vi "test.Zorder.vi"() -> ()   [LabVIEW 2020]
uses:
  WINUTIL.LLB/Window Rectangle.ctl
  <vilib>/Utility/miscctls.llb/LVRectTypeDef.ctl
  <userlib>/_OpenG.lib/comparison/comparison.llb/Boolean Changed__ogtk.vi
  WINUTIL.LLB/WINUTIL.lvlib
panel:
  in  "topmost":bool
  in  "stop":bool
  out "Array":T1[](array[typedef])
  out "Refnum out 2":T2[](array[typedef])
  out "window name 2":string[](array[string])
  out "Front Panel Window:Panel Bounds":T3
  out "window rect":T1
  out "window name":string
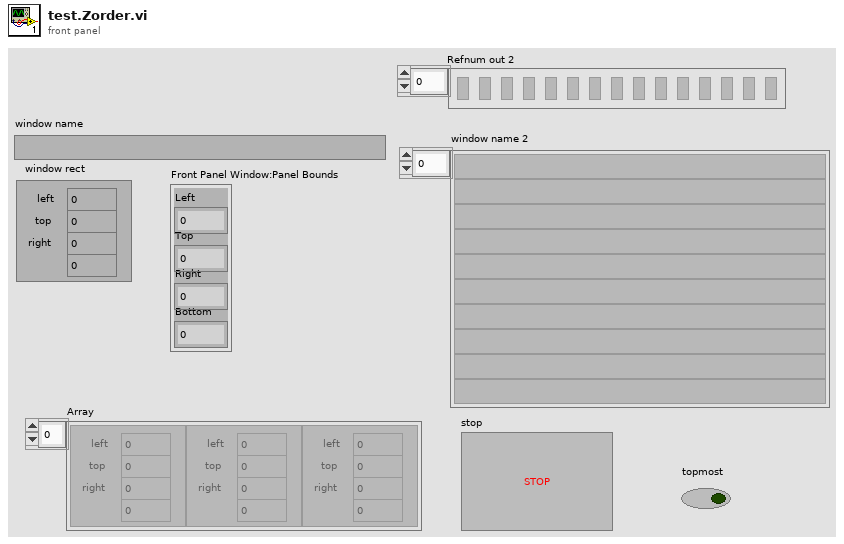
[diagram p1: front panel]
types:
  T1 = typedef "WINUTIL.lvlib/Window Rectangle.ctl" = cluster{"left":i16, "top":i16, "right":i16, "bottom":i16}
  T2 = typedef "WINUTIL.lvlib/Window Refnum" = refnum<k1>
  T3 = typedef "LVRectTypeDef.ctl" = cluster{"Left":i16, "Top":i16, "Right":i16, "Bottom":i16}
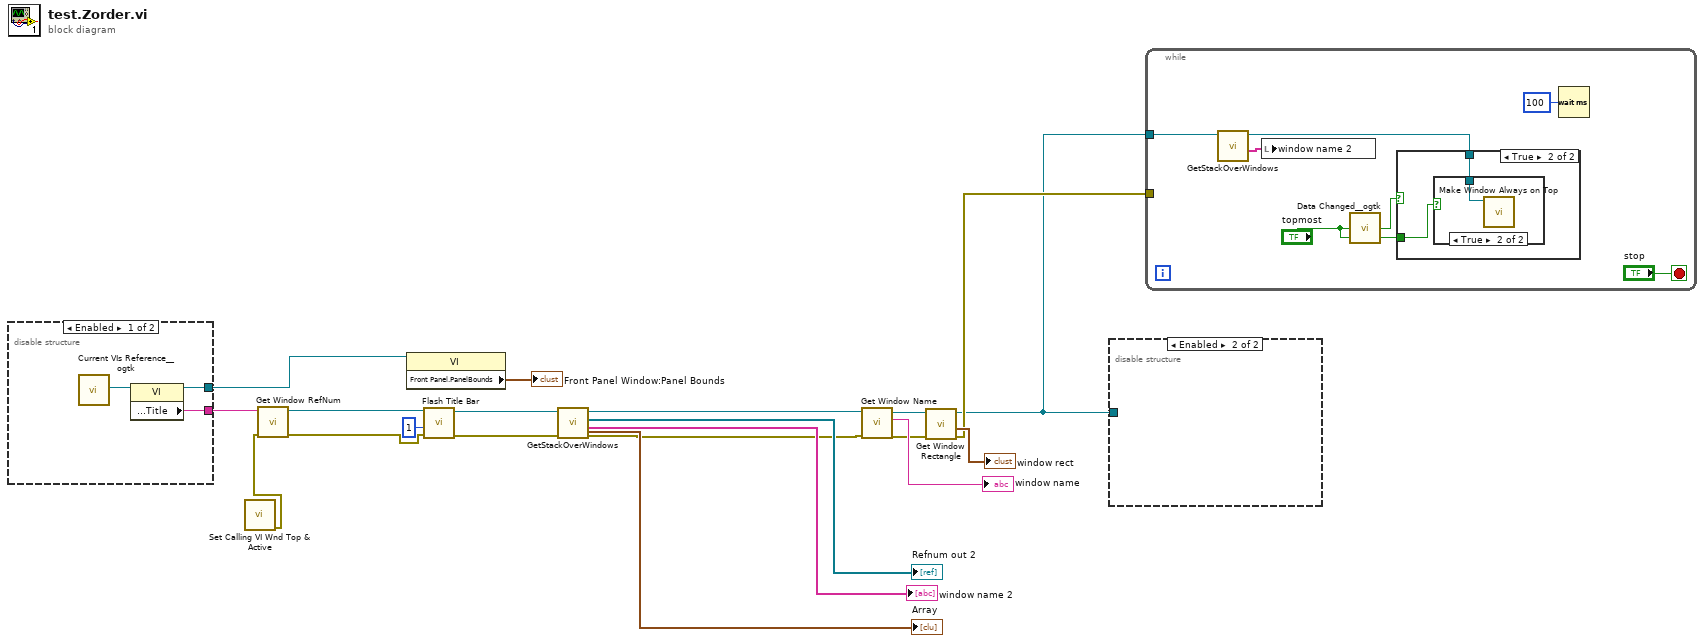
[diagram p0: block diagram]
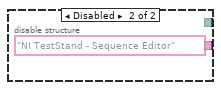
[diagram p2: hidden frame]
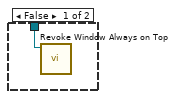
[diagram p4: hidden frame]
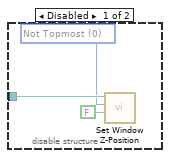
[diagram p5: hidden frame]
diagram:
  n1 = disable-structure shown="Enabled" {
    disable-tunnel: [w22 _] -> w16
    disable-tunnel: [w21 "NI TestStand - Sequence Editor" ("window name (\"\")")] -> w14
    frame Enabled {
      n2 = call <userlib>:"Current VIs Reference__ogtk.vi"() -> ("Current VI's reference"=w23:refnum<vi>)  [unwired: 5 in]
      n3 = property class="VI"(reference=w23) -> (reference out=w22:refnum<vi>, "Front Panel.Title"=w21:string)  [unwired: 1 in, 1 out]
    }
    frame Disabled {
    }
  }
  n4 = call "Set Calling VI Wnd Top & Active.vi"() -> ("Error Out"=w1:errorcluster)  [unwired: 11 in]
  n5 = call "Get Window RefNum.vi"("error in (no error)"=w1, "window name (\"\")"=w14) -> ("error out"=w5:errorcluster, "window refnum (NaWR)"=w8:T2)  [unwired: 6 in]
  n6 = property class="VI"(reference=w16) -> ("Front Panel.PanelBounds"=→"Front Panel Window:Panel Bounds":T3)  [unwired: 1 in, 2 out]
  n7 = call "Flash Title Bar.vi"("error in (no error)"=w5, "number of flashes (1)"=1, "window refnum (NaWR)"=w8) -> ("error out"=w4:errorcluster, "window refnum out"=w13:T2)  [unwired: 4 in]
  n8 = call "GetStackOverWindows.vi"("error in (no error)"=w4, "Refnum in"=w13) -> ("error out"=w3:errorcluster, "window name"=→"window name 2":string[], "Refnum out 2"=→"Refnum out 2":T2[], "Refnum out"=w12:T2, "Array"=→"Array":T1[])  [unwired: 5 in]
  n9 = call "Get Window Name.vi"("error in (no error)"=w3, "window refnum in (NaWR)"=w12) -> ("error out"=w2:errorcluster, "window name"=→"window name":string, "window refnum out"=w18:T2)  [unwired: 3 in]
  n10 = call "Get Window Rectangle.vi"("error in (no error)"=w2, "window refnum (NaWR)"=w18) -> ("error out"=w7:errorcluster, "window rect"=→"window rect":T1, "window refnum out"=w6:T2)  [unwired: 3 in]
  n11 = disable-structure shown="Enabled" {
    disable-tunnel: w6 -> [w27 _]
    frame Disabled {
      w26 = i16 0 items=["Not Topmost", "Topmost", "Top", "Bottom"] ("z-order position")
      n12 = call "Set Window Z-Position.vi"("activate? (T)"=FALSE, "z-order position"=w26, "window refnum"=w27) -> ()  [unwired: 3 in, 2 out]
    }
    frame Enabled {
    }
  }
  n13 = while {
    tunnel: w6 -> [w33]
    tunnel: w7 -> [_]
    stop <- "stop" stop-if-true
    n14 = call "GetStackOverWindows.vi"("Refnum in"=w33) -> ("window name"=w32:string[], "Refnum out"=w29:T2)  [unwired: 6 in, 3 out]
    n15 = local write "window name 2"(w32) -> ()
    n16 = call-poly <userlib>:"Data Changed__ogtk.vi"("Boolean"="topmost") -> ("Changed"=w30:bool)
    n17 = case shown="True" w30 {
      tunnel: w29 -> [_ w36]
      tunnel: "topmost" -> [_ w35]
      frame False {
      }
      frame True {
        n18 = case shown="True" w35 {
          tunnel: w36 -> [w37 w38]
          frame False {
            n19 = call "Revoke Window Always on Top.vi"("window refnum (NaWR)"=w37) -> ()  [unwired: 5 in, 2 out]
          }
          frame True {
            n20 = call "Make Window Always on Top.vi"("window refnum (NaWR)"=w38) -> ()  [unwired: 5 in, 2 out]
          }
        }
      }
    }
    n21 = Wait (ms)(milliseconds to wait=u32 100) -> ()  [unwired: 1 out]
  }
